vi "Analyse Break.vi"(8 "error in (no error)":errorcluster, 11 "Waveform in":dbl[](graph)) -> (0 "error out":errorcluster, 2 "Number of Peaks":i32, 3 "Peak Indexes":i32[](array[numeric]))   [LabVIEW 2019]
panel:
  out "Amplified Graph":dbl[](graph)
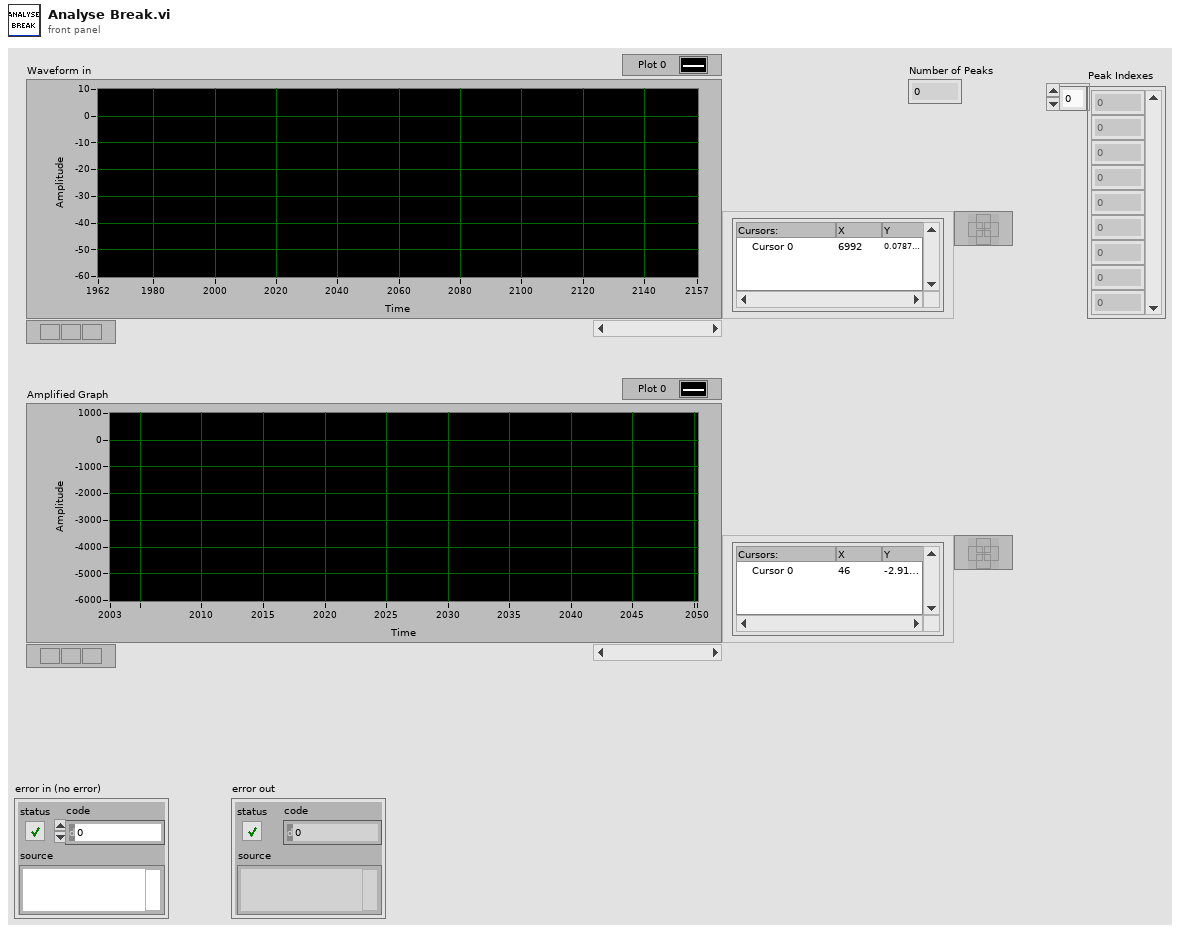
[diagram p1: front panel]
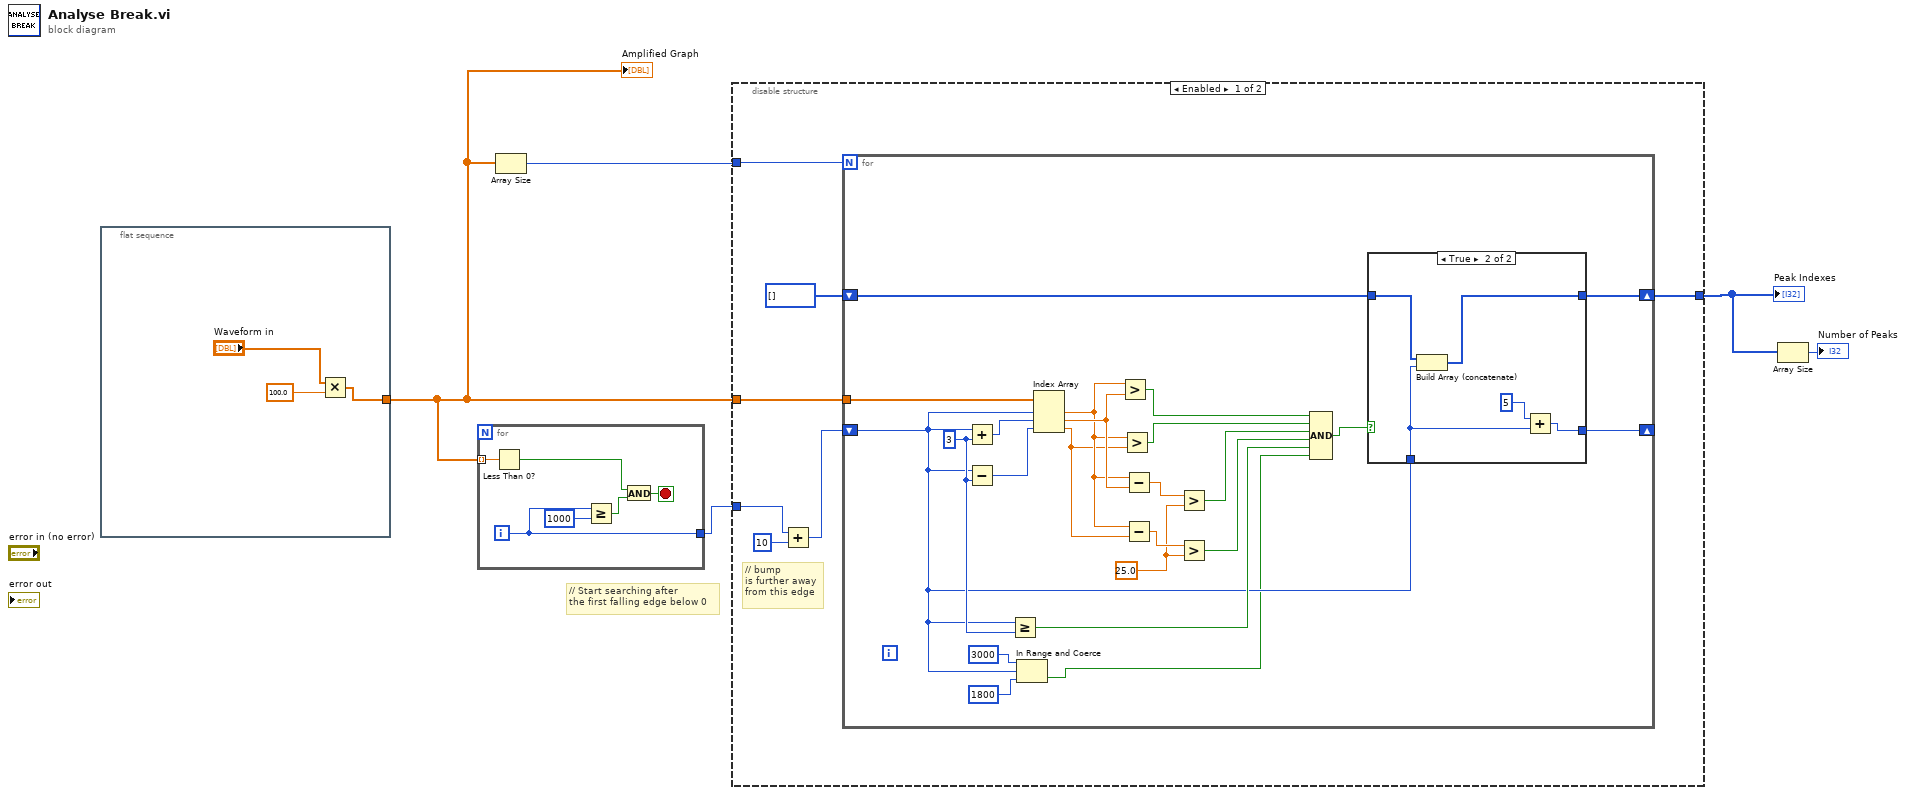
[diagram p0: block diagram]
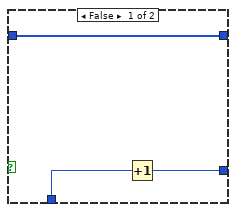
[diagram p2: hidden frame]
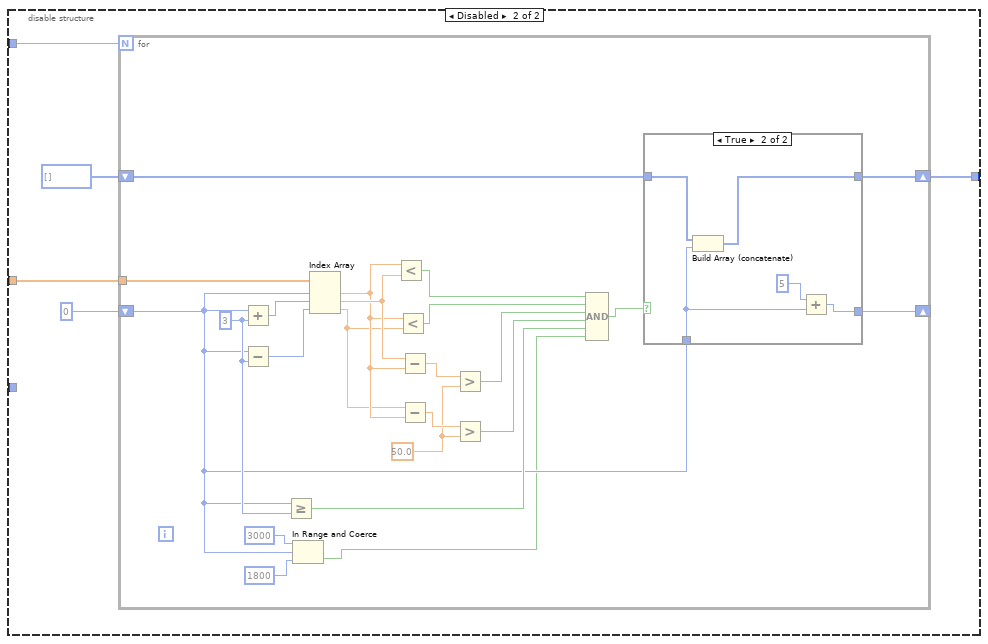
[diagram p3: hidden frame]
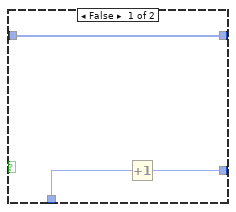
[diagram p4: hidden frame]
diagram:
  # "// Start searching after\nthe first falling edge below 0"
  n1 = flat-sequence {
    tunnel: [w6] -> w2
    frame #0 {
      n2 = Multiply(x="Waveform in", y=100.0) -> (x*y=w6:dbl[])
    }
  }
  n3 = for {
    tunnel: w2 -> [w14] mode=indexing
    tunnel: [w10] -> w1
    i -> [w10]
    stop <- w13 stop-if-true
    n4 = Less Than 0?(x=w14) -> (x < 0?=w12:bool)
    n5 = Greater Or Equal?(x=w10, y=1000) -> (x >= y?=w11:bool)
    n6 = And(x=w12, y=w11) -> (x .and. y?=w13:bool)
  }
  n7 = Array Size(array=w2) -> (size(s)=w5:i32)
  n8 = disable-structure shown="Enabled" {
    disable-tunnel: w2 -> [w21 w57]
    disable-tunnel: w5 -> [w20 w55]
    disable-tunnel: [w18 w53] -> w4
    disable-tunnel: w1 -> [w17 _]
    frame Enabled {
      # "// bump\nis further away\nfrom this edge"
      n9 = Add(x=w17, y=10) -> (x+y=w16:i32)
      n10 = for {
        N: w20 -> [_]
        tunnel: w21 -> [w44]
        shift-right: [w30] -> _
        shift-left: w16 -> [w25]
        shift-right: [w29] -> w18
        shift-left: i32[] [] -> [w28]
        w34 = 25.0 ("y")
        w27 = 3 ("y")
        n11 = Add(x=w25, y=w27) -> (x+y=w42:i32)
        n12 = Subtract(x=w25, y=w27) -> (x-y=w43:i32)
        n13 = Greater Or Equal?(x=w25, y=w27) -> (x >= y?=w26:bool)
        n14 = In Range and Coerce(upper limit=3000, x=w25, lower limit=1800 ("upper limit")) -> (In Range?=w22:bool)  [unwired: 1 out]
        n15 = Index Array(array=w44, index #1=w25, index #2=w42, index #3=w43) -> (element #1=w38:dbl, element #2=w39:dbl, element #3=w37:dbl)
        n16 = Greater?(x=w38, y=w39) -> (0:w41:bool)
        n17 = Greater?(x=w38, y=w37) -> (0:w40:bool)
        n18 = Subtract(x=w38, y=w39) -> (x-y=w36:dbl)
        n19 = Subtract(x=w38, y=w37) -> (x-y=w35:dbl)
        n20 = Greater?(x=w36, y=w34) -> (0:w33:bool)
        n21 = Greater?(x=w35, y=w34) -> (0:w32:bool)
        n22 = Compound Arithmetic op=AND(w41, w40, w33, w32, w26, w22) -> (w31:bool)
        n23 = case shown="True" w31 {
          tunnel: w25 -> [w47 w51]
          tunnel: [w46 w50] -> w30
          tunnel: [w45 w49] -> w29
          tunnel: w28 -> [w45 w48]
          frame False {
            n24 = Increment(x=w47) -> (x+1=w46:i32)
          }
          frame True {
            n25 = Build Array (concatenate)(w48, w51) -> (w49:i32[])
            n26 = Add(x=5, y=w51) -> (x+y=w50:i32)
          }
        }
      }
    }
    frame Disabled {
      n27 = for {
        N: w55 -> [_]
        tunnel: w57 -> [w80]
        shift-right: [w66] -> _
        shift-left: 0 -> [w61]
        shift-right: [w65] -> w53
        shift-left: i32[] [] -> [w64]
        w70 = 50.0 ("y")
        w63 = 3 ("y")
        n28 = Add(x=w61, y=w63) -> (x+y=w78:i32)
        n29 = Subtract(x=w61, y=w63) -> (x-y=w79:i32)
        n30 = Greater Or Equal?(x=w61, y=w63) -> (x >= y?=w62:bool)
        n31 = In Range and Coerce(upper limit=3000, x=w61, lower limit=1800 ("upper limit")) -> (In Range?=w58:bool)  [unwired: 1 out]
        n32 = Index Array(array=w80, index #1=w61, index #2=w78, index #3=w79) -> (element #1=w74:dbl, element #2=w75:dbl, element #3=w73:dbl)
        n33 = Less?(x=w74, y=w75) -> (x < y?=w77:bool)
        n34 = Less?(x=w74, y=w73) -> (x < y?=w76:bool)
        n35 = Subtract(x=w75, y=w74) -> (x-y=w72:dbl)
        n36 = Subtract(x=w73, y=w74) -> (x-y=w71:dbl)
        n37 = Greater?(x=w72, y=w70) -> (0:w69:bool)
        n38 = Greater?(x=w71, y=w70) -> (0:w68:bool)
        n39 = Compound Arithmetic op=AND(w77, w76, w69, w68, w62, w58) -> (w67:bool)
        n40 = case shown="True" w67 {
          tunnel: w61 -> [w83 w87]
          tunnel: [w82 w86] -> w66
          tunnel: [w81 w85] -> w65
          tunnel: w64 -> [w81 w84]
          frame False {
            n41 = Increment(x=w83) -> (x+1=w82:i32)
          }
          frame True {
            n42 = Build Array (concatenate)(w84, w87) -> (w85:i32[])
            n43 = Add(x=5, y=w87) -> (x+y=w86:i32)
          }
        }
      }
    }
  }
  "Peak Indexes" <- w4
  n44 = Array Size(array=w4) -> (size(s)=→"Number of Peaks":i32)
  "Amplified Graph" <- w2
